vi "ParentModuleTemplate.vi"(11 "Module Config":T2={"Name"="Direct Drive Control System", "Parent Q"=refnum, "Is Child?"=FALSE, "Index"=0, "Dirs"={"Root"=path "", "Config"=path "C:/ATE/Config", "Logs"=path "C:/ATE/Logs", "Reports"=path "C:/ATE/Reports", "App Data"=path "C:/ProgramData/MAIN"}}) -> ()   [LabVIEW 2016]
uses:
  <vilib>/KATE/Queues/Queue Utils.lvlib
  <vilib>/KATE/Module/Module Utils.lvlib
  <vilib>/KATE/Module/Public/Action - Window Tasks.ctl
  <vilib>/KATE/Scheduler/Scheduler.lvlib
  <vilib>/KATE/Event Log/Event Log.lvlib
  <vilib>/KATE/Module/Public/Error Report.ctl
  <vilib>/KATE/Files/File Utils.lvlib
  <vilib>/Utility/miscctls.llb/LVRowAndColumnUnsignedTypeDef.ctl
  Controls & Typedefs/Log File Info.ctl
  Utils/Config/Save Control States/Save Control - Action.ctl
  <vilib>/KATE/Queues/Q.Element.ctl
  <vilib>/KATE/Module/Module Config.ctl
  <vilib>/KATE/Module/Public/SW Version Info.ctl
  <vilib>/KATE/Module/Module.Working Dirs.ctl
panel:
  in  "Main UI Tab":enum32{"Operate", "Maint"}(tab)
  in  "Main Ctrl Tab":enum32{"Page 1", "Page 2"}(tab)
  in  "Control1":bool
  in  "Test Name":string="TestX" caption="(Report name)"
  in  "Operator":string
  out "Rev":string="v0.0.1"
  out "Simulate Indication":string="Simulating Instruments"
  out "Error":bool
  out "Title":string="App Name"
  in  "Data Tab":T1(tab)
  in  "Setup Control1":bool
  in  "Log Interval(s)":dbl=1.0
  in  "Open Log Folder":bool
  out "Report File Name":string
  out "Data Log":string[][](table)
  in  "Equipment List":string[][](table)=[["Function Generator", "", "", "", ""], ["", "", "", "", ""], ["", "", "", "", ""], ["", "", "", "", ""], ["", "", "", "", ""]]
  in  "Reset":bool
  out "Status":string
  out "Test Ctrl Tab":enum32{"Idle", "Running", "Completed"}(tab)
  in  "Start":bool
  out "Status Duration(s)":dbl caption="Duration(s)" format="%.1f"
  out "Status Elapsed(s)":dbl caption="Elapsed(s)" format="%.1f"
  out "Test Running":bool
  out "Progress":dbl(slide) scale=0.0..1.0
  in  "Abort":bool
  in  "Test Reset":bool
  in  "Simulate En":bool
  in  "Exit":bool
  in  "Show Block Diagram":bool
  in  "Leave Maint":bool
  in  "Maint":bool
  in  "SW Rev":T4={"AppName"="App Name", "Company"="Company Name", "Version"="0.0.1", "Date"="xx/xx/xx"}
  # "Company Icon"
  # "Test Info"
  # "Put controls here that you want \nto be always visible"
  # "Put test setup controls here"
  # "This si a subpanel to a child VI that controls the instrument"
  # "Function Generator\nInternal Memory Status"
  # "<Update Version and save as default values>"
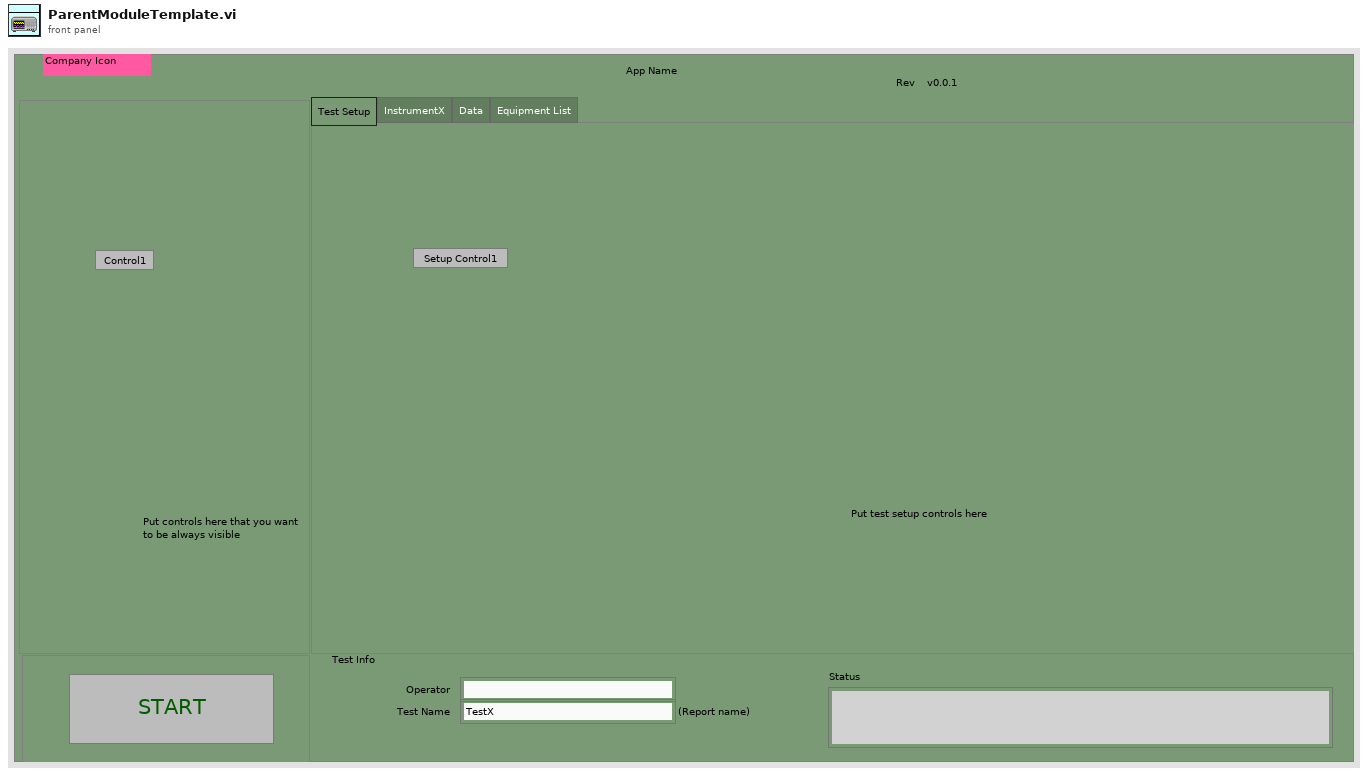
[diagram p1: front panel]
types:
  T1 = enum32{"Test Setup", "InstrumentX", "Data", "Equipment List"}
  T2 = typedef "KATE_Lib.lvlib/Module Utils.lvlib/Module Config.ctl" = cluster{"Name":string, "Parent Q":refnum<queue>, "Is Child?":bool, "Index":i32, "Dirs":T3}
  T3 = typedef "KATE_Lib.lvlib/Module Utils.lvlib/Module.Working Dirs.ctl" = cluster{"Root":path, "Config":path, "Logs":path, "Reports":path, "App Data":path}
  T4 = typedef "KATE_Lib.lvlib/Module Utils.lvlib/SW Version Info.ctl" = cluster{"AppName":string, "Company":string, "Version":string, "Date":string}
  T5 = typedef "KATE_Lib.lvlib/Module Utils.lvlib/Module Sys Info.ctl" = cluster{"Main Q":refnum<queue>, "Exe":bool, "SW Rev":T6, "Self Ref":refnum<vi>, "Main Tab":refnum<vi>, "Pane":refnum<vi>, "Stop":cluster{"Ref":refnum<event-registration>, "Event":refnum<user-event>}, "Cfg":T2, "Services":cluster{"Name":string, "vi ref":refnum<vi>}[]}
  T6 = typedef "KATE_Lib.lvlib/Module Utils.lvlib/Module.SW Version Info.ctl" = cluster{"AppName":string, "Company":string, "Version":string, "Date":string}
  T7 = typedef "KATE_Lib.lvlib/Module Utils.lvlib/Action - Window Tasks.ctl" = enum16{"Resize()", "Show Panel(Bool)", "Show Scroll Bars(Bool)", "Dock to SubPanel(SubPanel Ref)", "Undock from SubPanel()", "Return to SubPanel()", "Go To Maint Tab()", "Show Maint Tab(Bool)", "Open Block Diagram()"}
  T8 = cluster{"Test Start(s)":dbl, "StepStart(s)":dbl, "Running":bool}
  T9 = typedef "Save Control - Action.ctl" = enum16{"Read", "Save", "Add Single Ctrl", "Add Mult Ctrls", "Restore"}
  T10 = enum8{"Enabled", "Disabled", "Disabled and Grayed Out"}
  T11 = typedef "LVRowAndColumnUnsignedTypeDef.ctl" = cluster{"Row":u32, "Column":u32}
  T12 = typedef "Log File Info.ctl" = cluster{"Log Name":string, "Initialized":bool, "Cmt Flag":bool, "Open":bool, "FileRef":refnum<k34>}
  T13 = enum16{"open", "open or create", "create or replace", "create", "open (read-only)"}
  T14 = enum16{"Top Left", "Top Right", "Bottom Left", "Bottom Right"}
  T15 = cluster{"Test State":cluster{"Test Start(s)":dbl, "StepStart(s)":dbl, "Running":bool}, "Data Table":string[][], "Log":T12}
  T16 = typedef "KATE_Lib.lvlib/Module Utils.lvlib/Error Report.ctl" = cluster{"Cnt":i32, "Recent Error":errorcluster}
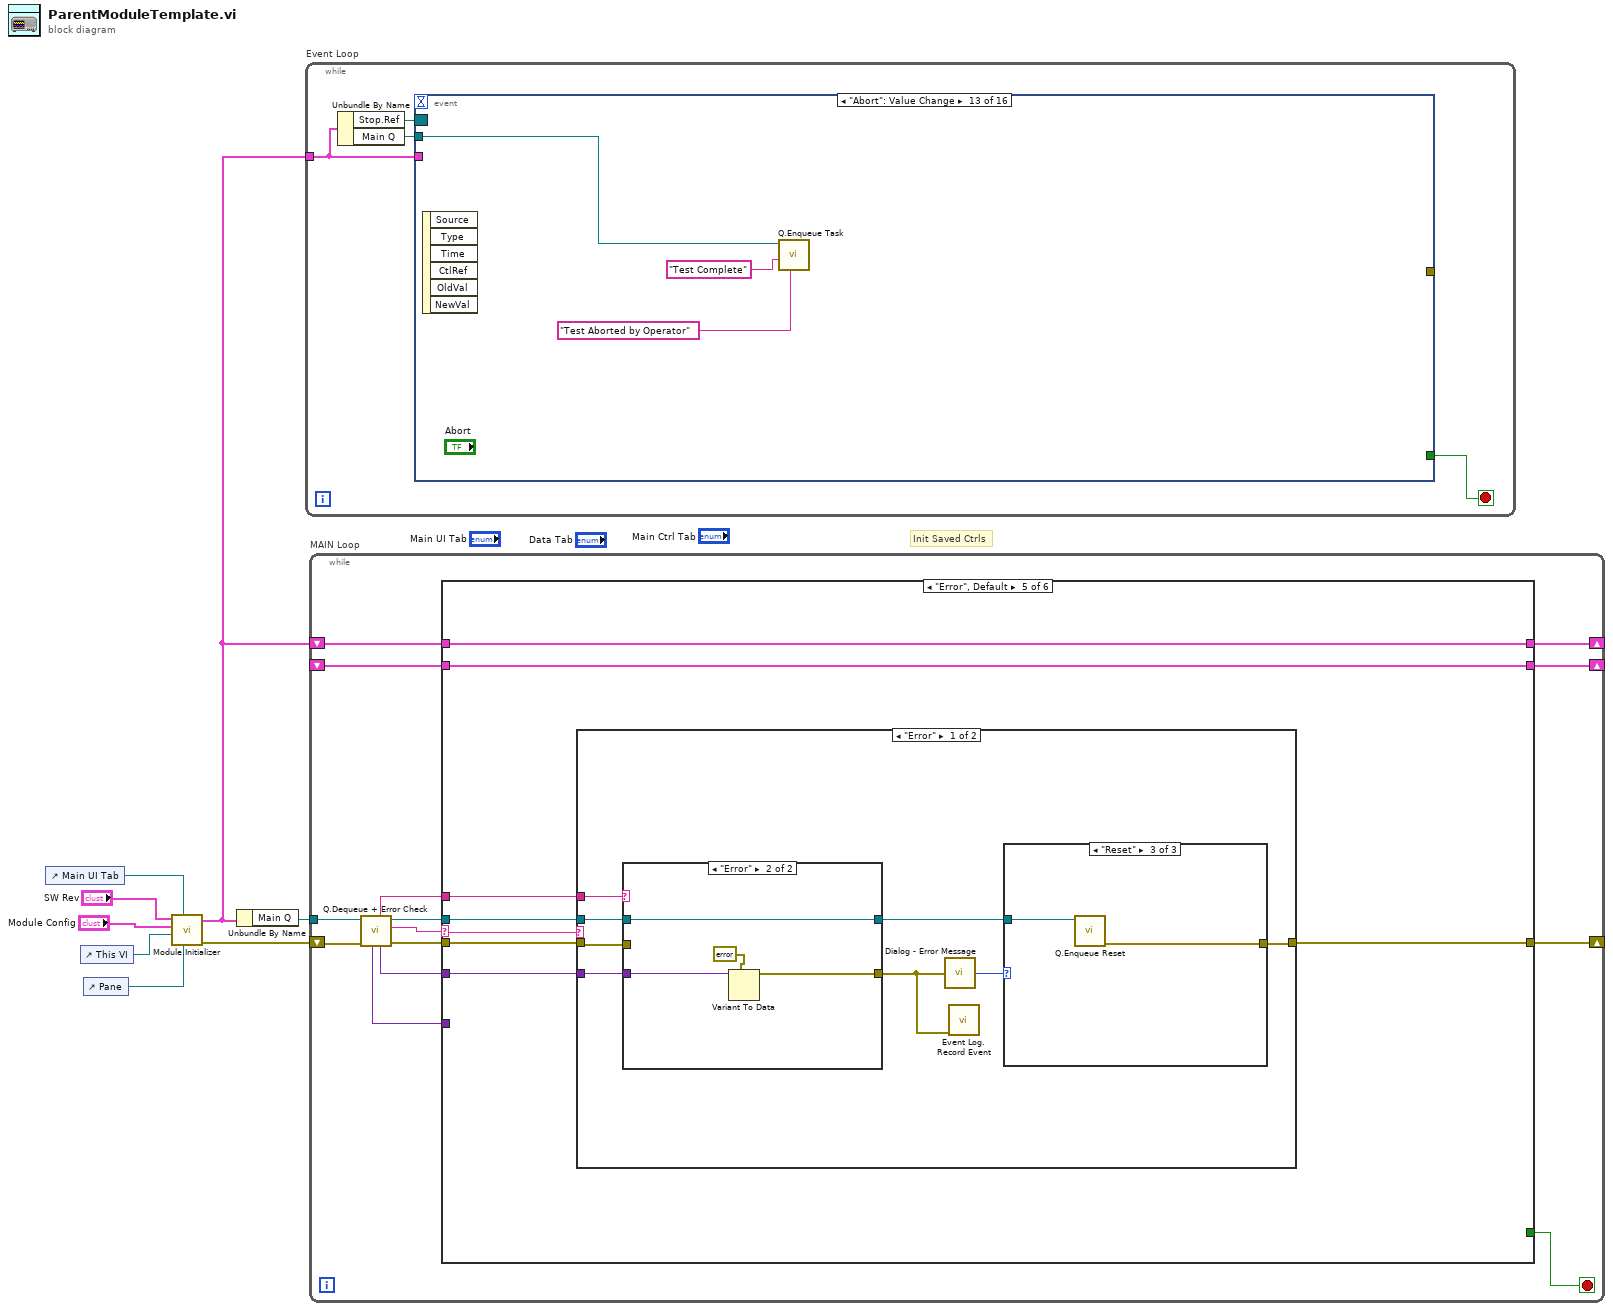
[diagram p0: block diagram]
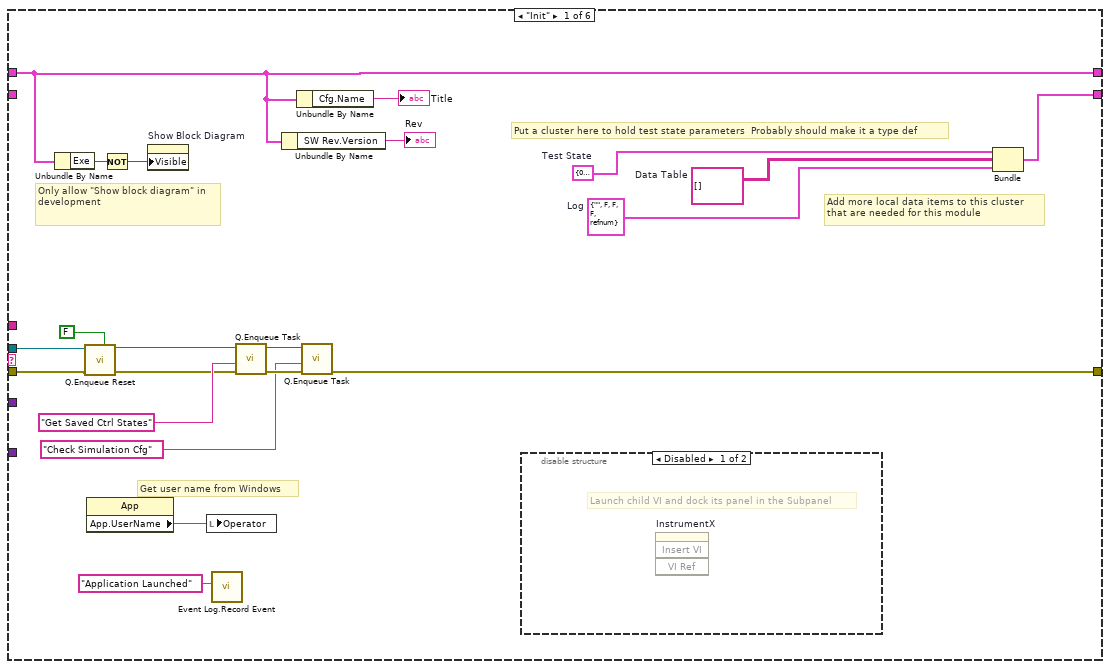
[diagram p2: hidden frame]
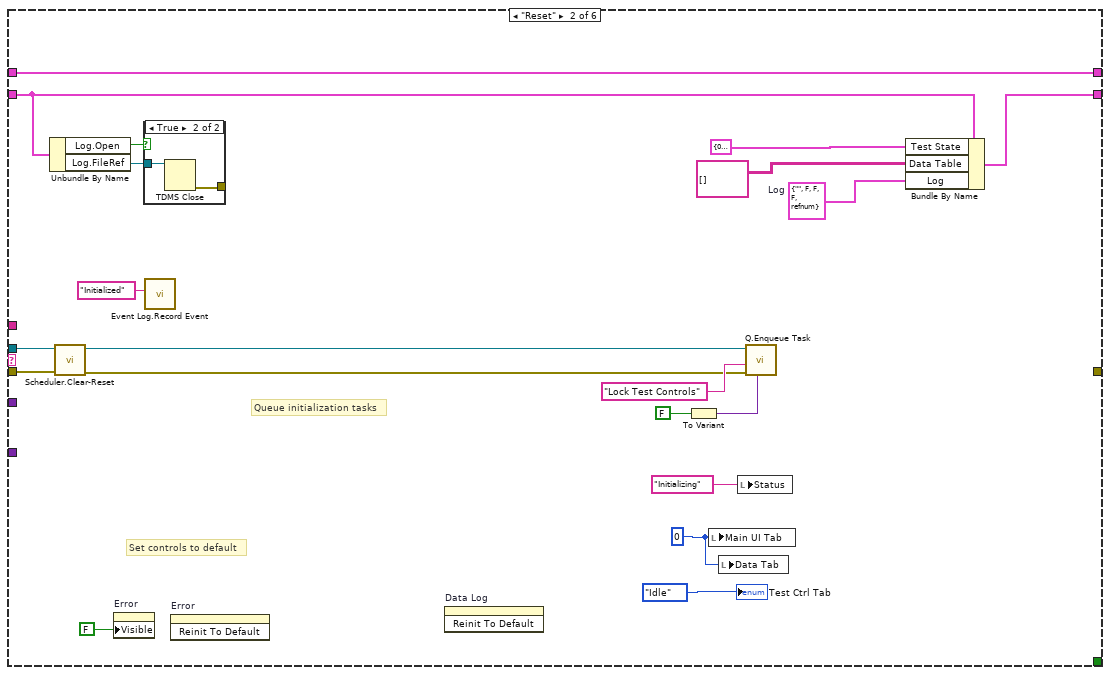
[diagram p4: hidden frame]
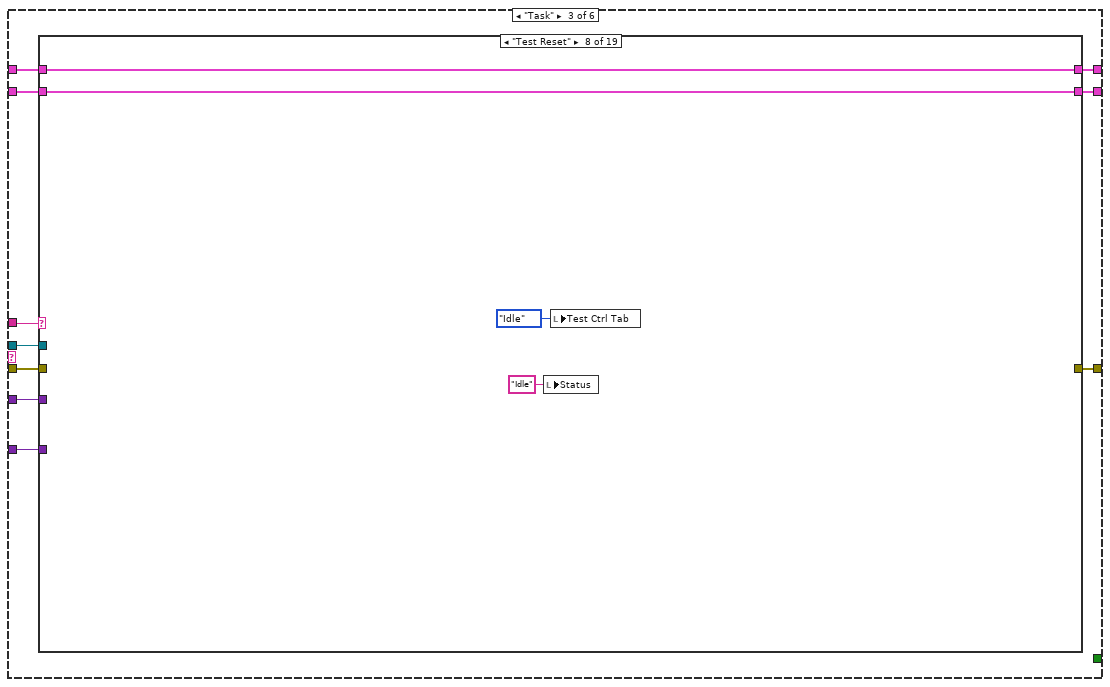
[diagram p6: hidden frame]
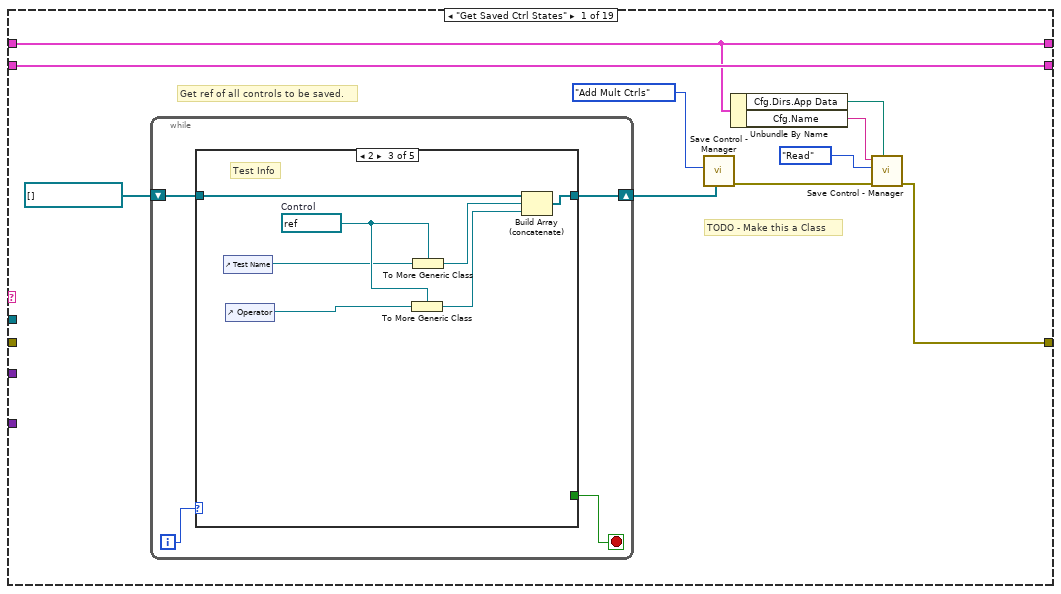
[diagram p7: hidden frame]
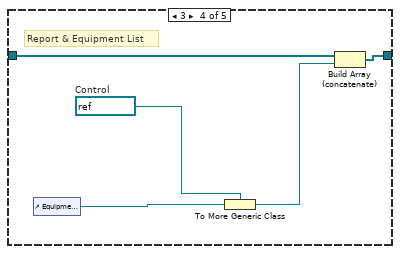
[diagram p10: hidden frame]
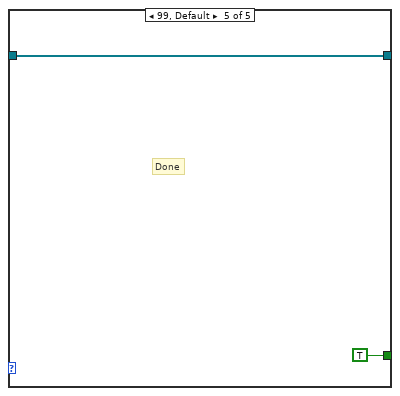
[diagram p11: hidden frame]
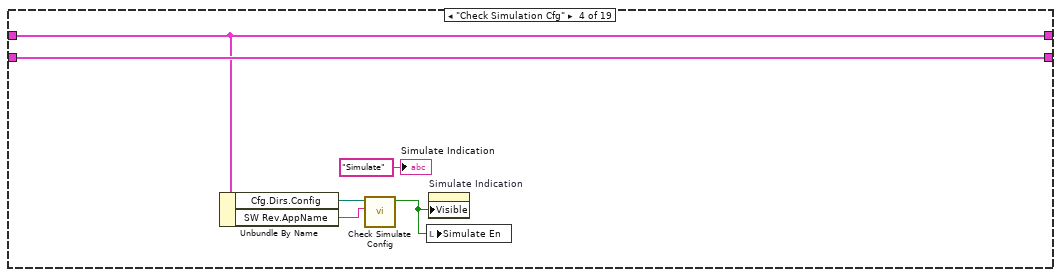
[diagram p14: hidden frame]
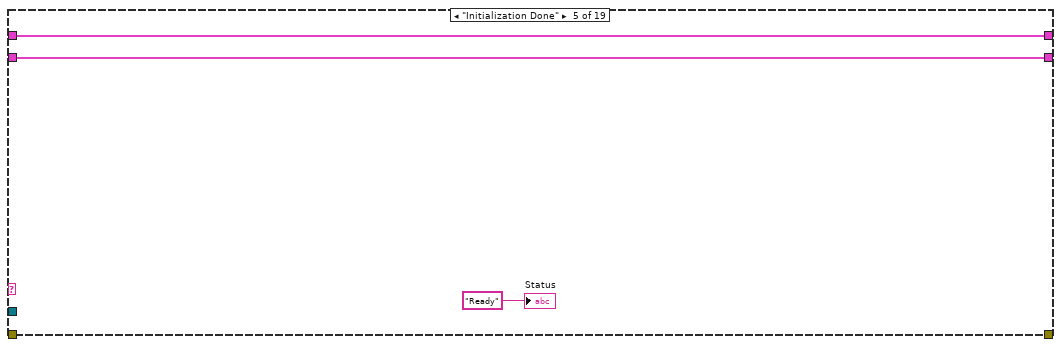
[diagram p15: hidden frame]
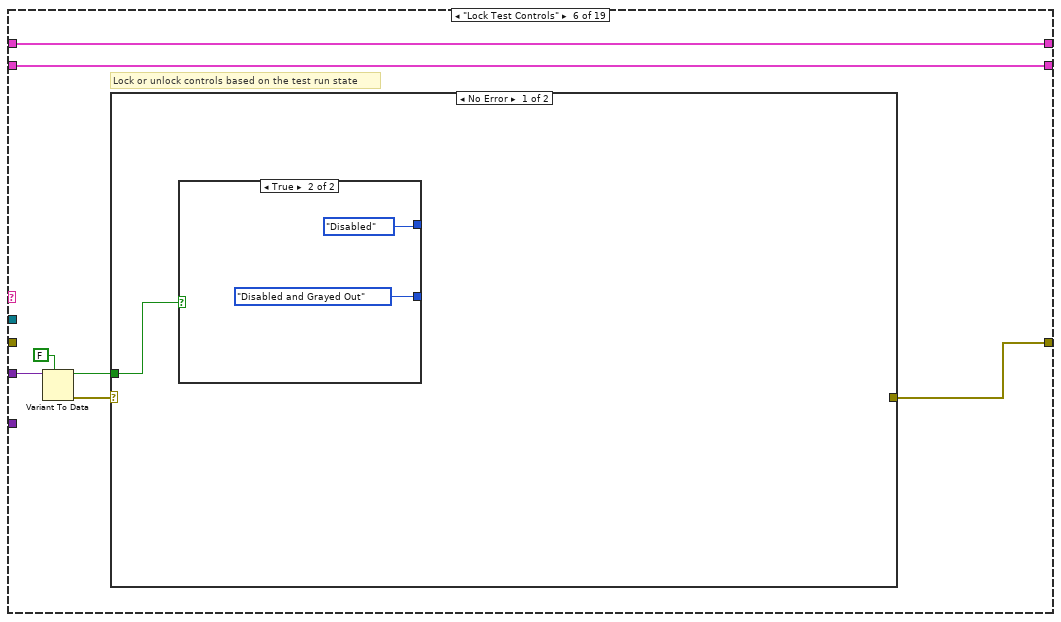
[diagram p16: hidden frame]
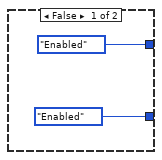
[diagram p17: hidden frame]
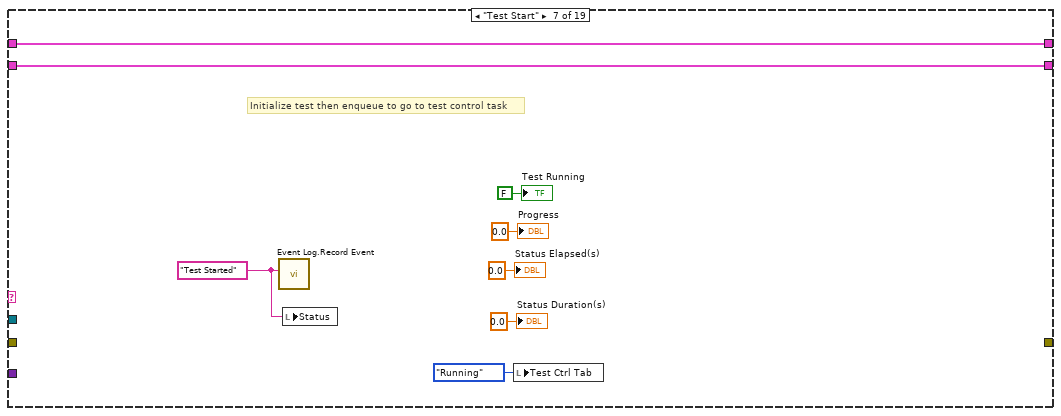
[diagram p19: hidden frame]
diagram:
  # "Init Saved Ctrls"
  n1 = control-ref of="Main UI Tab"() -> (w5:refnum<vi>)
  n2 = control-ref of="This VI"() -> (w4:refnum<vi>)
  n3 = control-ref of="Pane"() -> (w3:refnum<vi>)
  n4 = call <vilib>:"Module.Initializer.vi"("Pane"=w3, "Main Tab"=w5, "Self Ref"=w4, "Module Config"="Module Config", "SW Rev"="SW Rev") -> ("error out"=w8:errorcluster, "Sys"=w7:T5)  [unwired: 5 in]
  n5 = Unbundle By Name(w7) -> ("Main Q"=w6:refnum<queue>)
  n6 = while "Event Loop" {
    tunnel: w7 -> [w11]
    stop <- w12 stop-if-true
    n7 = Unbundle By Name(w11) -> ("Stop.Ref"=w10:refnum<event-registration>, "Main Q"=w9:refnum<queue>)
    n8 = event shown="[12] \"Abort\": Value Change" {
      selector: w10 -> [_ _ _ _ _ _ _ _ _ _ _ _ _ _ _ _]
      dyn-events: _ -> [_ _ _ _ _ _ _ _ _ _ _ _ _ _ _ _]
      timeout: _ -> [_ _ _ _ _ _ _ _ _ _ _ _ _ _ _ _]
      tunnel: [w16 TRUE _ _ _ _ _ w40 TRUE _ _ _ _ _ _ _] -> w12
      tunnel: w11 -> [w15 _ _ _ _ _ _ w38 _ w65 _ _ _ _ w81 _]
      tunnel: w9 -> [w18 w28 w30 w32 w34 w36 _ w39 _ _ w66 w71 w76 w78 _ w82]
      tunnel: [_ _ _ _ _ _ _ _ _ _ _ _ _ _ w79 _] -> _
      event Panel Close? {
        n9 = event-data() -> ()  [unwired: 1 in, 4 out]
        n10 = Unbundle By Name(w15) -> ("Exe"=w13:bool, "Cfg.Is Child?"=w14:bool)
        n11 = case shown="False" w14 {
          tunnel: w18 -> [w22 w25]
          tunnel: [w20 TRUE] -> w17
          tunnel: [TRUE FALSE] -> w16
          tunnel: [_ w23] -> _
          tunnel: w13 -> [w19 _]
          frame False {
            # "Parent - Exit"
            n12 = call <vilib>:"Q.Enqueue Exit.vi"("Q In"=w22) -> ()  [unwired: 9 in, 2 out]
            n13 = Not(x=w19) -> (.not. x?=w20:bool)
          }
          frame True {
            # "Child - Hide Panel"
            n14 = call <vilib>:"Q Window Task.vi"("Action"=Action_-_Window_Tasks."Return to SubPanel()", "Q In"=w25) -> ("error out"=w23:errorcluster)  [unwired: 8 in, 1 out]
          }
        }
        n15 = event-data("Discard?"=w17) -> ()  [unwired: 1 in, 1 out]
      }
      event "Exit": Value Change {
        n16 = event-data() -> ()  [unwired: 1 in, 6 out]
        n17 = call <vilib>:"Q.Enqueue Exit.vi"("Q In"=w28) -> ()  [unwired: 9 in, 2 out]
      }
      event "Reset": Value Change {
        n18 = event-data() -> ()  [unwired: 1 in, 6 out]
        n19 = call <vilib>:"Q.Enqueue Reset.vi"("Q In"=w30) -> ()  [unwired: 9 in, 2 out]
      }
      event Panel Resize {
        n20 = event-data() -> ()  [unwired: 1 in, 8 out]
        n21 = call <vilib>:"Q Window Task.vi"("Action"=Action_-_Window_Tasks."Resize()", "Q In"=w32) -> ()  [unwired: 8 in, 2 out]
      }
      event "Show Block Diagram": Value Change {
        n22 = event-data() -> ()  [unwired: 1 in, 6 out]
        n23 = call <vilib>:"Q Window Task.vi"("Action"=Action_-_Window_Tasks."Open Block Diagram()", "Q In"=w34) -> ()  [unwired: 8 in, 2 out]
      }
      event "Maint": Value Change {
        n24 = event-data() -> ()  [unwired: 1 in, 6 out]
        n25 = call <vilib>:"Q Window Task.vi"("Action"=Action_-_Window_Tasks."Go To Maint Tab()", "Q In"=w36) -> ()  [unwired: 8 in, 2 out]
      }
      event "Leave Maint": Value Change {
        n26 = event-data() -> ()  [unwired: 1 in, 6 out]
        n27 = local write "Main UI Tab"(0) -> ()
      }
      event Menu Selection (User) {
        n28 = event-data() -> ("ItemTag"=w41:string)  [unwired: 1 in, 6 out]
        n29 = case shown="Default" w41 {
          tunnel: [_ TRUE _ _ _ _ _] -> w40
          tunnel: w39 -> [_ w42 _ w45 _ _ _]
          tunnel: [_ _ w44 _ w46 _ w51] -> _
          tunnel: w38 -> [_ _ _ _ w47 w50 w60]
          frame Default {
          }
          frame "Exit" {
            n30 = call <vilib>:"Q.Enqueue Exit.vi"("Q In"=w42) -> ()  [unwired: 9 in, 2 out]
          }
          frame "Show Event Log" {
            n31 = call <vilib>:"Event Log.Show.vi"() -> ("error out"=w44:errorcluster)  [unwired: 11 in]
          }
          frame "Reset" {
            n32 = call <vilib>:"Q.Enqueue Reset.vi"("Q In"=w45) -> ()  [unwired: 9 in, 2 out]
          }
          frame "Open Log Folder" {
            n33 = Unbundle By Name(w47) -> ("Cfg.Dirs.Logs"=w48:path)
            n34 = call <vilib>:"File.Open File or Folder.vi"("Path"=w48) -> ("Error Out"=w46:errorcluster)  [unwired: 10 in]
          }
          frame "Help.About" {
            n35 = Unbundle By Name(w50) -> ("SW Rev"=w49:T6)
            n36 = call "Help.About.vi"("SW Version"=w49) -> ()  [unwired: 11 in]
          }
          frame "Help.User Manual" {
            n37 = Unbundle By Name(w60) -> ("SW Rev.AppName"=w59:string)
            n38 = call <vilib>:"Application Directory.vi"() -> ("Application Directory"=w55:path)
            n39 = Build Path(base path=w55, name or relative path="Documentation") -> (appended path=w54:path)
            n40 = Concatenate Strings("User Manual, ", w59, ".pdf") -> (w53:string)
            n41 = Build Path(base path=w54, name or relative path=w53) -> (appended path=w52:path)
            n42 = call <vilib>:"File.Open File or Folder.vi"("Path"=w52) -> ("Error Out"=w51:errorcluster)  [unwired: 10 in]
          }
        }
      }
      event User Event {
        n43 = event-data() -> ()  [unwired: 1 in, 5 out]
      }
      event "Simulate En": Value Change {
        n44 = event-data() -> ()  [unwired: 1 in, 6 out]
        n45 = Unbundle By Name(w65) -> ("Cfg.Dirs.Config"=w64:path, "SW Rev.AppName"=w63:string)
        n46 = call "Save Simulate Config.vi"("Simulate"="Simulate En", "App Name"=w63, "Config Folder"=w64) -> ()  [unwired: 8 in, 1 out]
        n47 = property on="Simulate Indication" class="Str"("Visible"="Simulate En") -> ()  [unwired: 2 in, 2 out]
      }
      event "Control1": Value Change {
        # "This code is a template for how to handle a control event.  \nEnque one or more tasks to handle the control change event"
        n48 = event-data() -> ()  [unwired: 1 in, 6 out]
        n49 = To Variant(anything="Control1") -> (Variant=w68:variant)
        n50 = call <vilib>:"Q.Enqueue Task.vi"("Data1"=w68, "Task Name"="Control1", "Q In"=w66) -> ()  [unwired: 7 in, 2 out]
      }
      event "Setup Control1": Value Change {
        # "This code is a template for how to handle a control event.  \nEnque one or more tasks to handle the control change event"
        n51 = event-data() -> ()  [unwired: 1 in, 6 out]
        n52 = To Variant(anything="Setup Control1") -> (Variant=w72:variant)
        n53 = call <vilib>:"Q.Enqueue Task.vi"("Data1"=w72, "Task Name"="Setup Control1", "Q In"=w71) -> ()  [unwired: 7 in, 2 out]
      }
      event "Abort": Value Change {
        n54 = event-data() -> ()  [unwired: 1 in, 6 out]
        n55 = call <vilib>:"Q.Enqueue Task.vi"("Data1"="Test Aborted by Operator" ("Message"), "Task Name"="Test Complete", "Q In"=w76) -> ()  [unwired: 7 in, 2 out]
      }
      event "Test Reset": Value Change {
        n56 = event-data() -> ()  [unwired: 1 in, 6 out]
        n57 = call <vilib>:"Q.Enqueue Task.vi"("Task Name"="Test Reset", "Q In"=w78) -> ()  [unwired: 8 in, 2 out]
      }
      event "Open Log Folder": Value Change {
        n58 = event-data() -> ()  [unwired: 1 in, 6 out]
        n59 = Unbundle By Name(w81) -> ("Cfg.Dirs.Reports"=w80:path)
        n60 = call <vilib>:"File.Open File or Folder.vi"("Path"=w80) -> ("Error Out"=w79:errorcluster)  [unwired: 10 in]
      }
      event "Start": Value Change {
        n61 = event-data() -> ()  [unwired: 1 in, 6 out]
        n62 = call <vilib>:"Q.Enqueue Task.vi"("Task Name"="Test Start", "Q In"=w82) -> ()  [unwired: 8 in, 2 out]
      }
    }
  }
  n63 = while "MAIN Loop" {
    shift-right: [w93] -> _
    shift-left: w8 -> [w91]
    shift-right: [w94] -> _
    shift-left: _ -> [w97]
    shift-right: [w95] -> _
    shift-left: w7 -> [w96]
    tunnel: w6 -> [w90]
    stop <- w84 stop-if-true
    n64 = call <vilib>:"Q.Dequeue + Error Check.vi"("Error In"=w91, "Q In"=w90) -> ("error out"=w92:errorcluster, "Cmd"=w89:string, "Q Out"=w88:refnum<queue>, "Data1"=w87:variant, "Sub"=w85:string, "Data2"=w86:variant)  [unwired: 4 in]
    n65 = case shown="\"Error\", Default" w89 {
      selector: w89 -> [_ _ _ _ w440 _]
      tunnel: w97 -> [_ w125 w149 w430 w442 w469]
      tunnel: w96 -> [w106 w131 w150 w431 w443 w471]
      tunnel: [w106 w131 w148 w429 w443 w471] -> w95
      tunnel: [w102 w133 w147 w428 w442 w469] -> w94
      tunnel: [w101 _ w141 w423 w441 w477] -> w93
      tunnel: w92 -> [w117 w137 w143 w424 w438 _]
      tunnel: w88 -> [w118 w138 w144 w425 w436 _]
      tunnel: w87 -> [_ _ w145 w426 w439 _]
      tunnel: w86 -> [_ _ w142 w422 _ _]
      tunnel: w85 -> [_ _ w146 w427 w437 _]
      tunnel: [_ _ _ _ _ TRUE] -> w84
      frame "Init" {
        w100 = T8 {"Test Start(s)"=0.0, "StepStart(s)"=0.0, "Running"=FALSE}  # Test State
        w108 = T12 {"Log Name"="", "Initialized"=FALSE, "Cmt Flag"=FALSE, "Open"=FALSE, "FileRef"=refnum}  # Log
        w112 = string[][] []  # Data Table
        # "Add more local data items to this cluster \nthat are needed for this module"
        # "Put a cluster here to hold test state parameters  Probably should make it a type def"
        # "Get user name from Windows"
        # "Only allow \"Show block diagram\" in development"
        n66 = Unbundle By Name(w106) -> ("Exe"=w115:bool)
        n67 = call <vilib>:"Q.Enqueue Reset.vi"("Top of Q(T)"=FALSE ("Flush Q"), "Error In"=w117, "Q In"=w118) -> ("error out"=w98:errorcluster, "Q Out"=w99:refnum<queue>)  [unwired: 7 in]
        n68 = property class="App"() -> ("App.UserName"=w109:string)  [unwired: 2 in, 2 out]
        n69 = Not(x=w115) -> (.not. x?=w114:bool)
        n70 = property on="Show Block Diagram" class="Bool"("Visible"=w114) -> ()  [unwired: 2 in, 2 out]
        n71 = local write "Operator"(w109) -> ()
        n72 = call <vilib>:"Event Log.Record Event.vi"("Message"="Application Launched") -> ()  [unwired: 10 in, 1 out]
        n73 = call <vilib>:"Q.Enqueue Task.vi"("Error In"=w98, "Task Name"="Get Saved Ctrl States", "Q In"=w99) -> ("error out"=w104:errorcluster, "Q Out"=w105:refnum<queue>)  [unwired: 7 in]
        n74 = Unbundle By Name(w106) -> ("SW Rev.Version"=→"Rev":string)
        n75 = Unbundle By Name(w106) -> ("Cfg.Name"=→"Title":string)
        n76 = call <vilib>:"Q.Enqueue Task.vi"("Error In"=w104, "Task Name"="Check Simulation Cfg", "Q In"=w105) -> ("error out"=w101:errorcluster)  [unwired: 7 in, 1 out]
        n77 = disable-structure shown="Disabled" {
          frame Disabled {
            # "Launch child VI and dock its panel in the Subpanel"
            n78 = invoke on="InstrumentX" class="SubPnl" method="Insert VI"() -> ()  [unwired: 4 in, 4 out]
          }
          frame Enabled {
          }
        }
        n79 = Bundle("Test State"=w100, "Data Table"=w112, "Log"=w108) -> (w102:T15)  [unwired: 1 in]
      }
      frame "Reset" {
        w126 = T12 {"Log Name"="", "Initialized"=FALSE, "Cmt Flag"=FALSE, "Open"=FALSE, "FileRef"=refnum}  # Log
        w134 = 0
        # "Set controls to default"
        # "Queue initialization tasks"
        n80 = Unbundle By Name(w125) -> ("Log.Open"=w123:bool, "Log.FileRef"=w124:refnum<k34>)
        n81 = call <vilib>:"Scheduler.Clear-Reset.vi"("error in"=w137, "Q In"=w138) -> ("error out"=w120:errorcluster, "Q Out"=w119:refnum<queue>)  [unwired: 8 in]
        n82 = property on="Error" class="Bool (strict)"("Visible"=FALSE) -> ()  [unwired: 2 in, 2 out]
        n83 = case shown="True" w123 {
          tunnel: w124 -> [_ w140]
          tunnel: [_ w139] -> _
          frame False {
          }
          frame True {
            n84 = TDMS Close(11:w140) -> (0:w139:errorcluster)  [unwired: 1 in, 1 out]
          }
        }
        n85 = call <vilib>:"Event Log.Record Event.vi"("Message"="Initialized") -> ()  [unwired: 10 in, 1 out]
        n86 = invoke on="Error" class="Bool (strict)" method="Reinit To Default"() -> ()  [unwired: 3 in, 3 out]
        n87 = invoke on="Data Log" class="Tbl (strict)" method="Reinit To Default"() -> ()  [unwired: 3 in, 3 out]
        n88 = To Variant(anything=FALSE) -> (Variant=w129:variant)
        n89 = local write "Main UI Tab"(w134) -> ()
        n90 = local write "Data Tab"(w134) -> ()
        n91 = local write "Status"("Initializing" ("Status")) -> ()
        n92 = call <vilib>:"Q.Enqueue Task.vi"("Data1"=w129, "Error In"=w120, "Task Name"="Lock Test Controls", "Q In"=w119) -> ()  [unwired: 6 in, 2 out]
        n93 = Bundle By Name(cluster=w125, "Test State"=T8 {"Test Start(s)"=0.0, "StepStart(s)"=0.0, "Running"=FALSE}, "Data Table"=string[][] [], "Log"=w126) -> (w133:T15)
        "Test Ctrl Tab" <- enum32{"Idle", "Running", "Completed"}."Idle" ("Test Ctrl Tab")
      }
      frame "Task" {
        n94 = case shown="\"Test Reset\"" w146 {
          selector: w146 -> [_ _ _ _ _ _ _ _ _ _ _ _ _ _ _ _ _ _ w417]
          tunnel: w150 -> [w153 w182 w184 w185 w193 w200 w214 w218 w220 w228 w244 w256 w301 w334 w371 w381 w388 w391 w418]
          tunnel: w149 -> [w160 w181 w183 w190 w192 w199 w213 w217 w219 w227 w233 w258 w299 w331 w366 w380 w387 w392 w419]
          tunnel: [w153 w182 w184 w185 w193 w200 w214 w218 w220 w228 w244 w256 w301 w334 w371 w381 w388 w391 w418] -> w148
          tunnel: [w160 w181 w183 w190 w192 w199 w213 w217 w219 w227 w238 w257 w298 w331 w366 w379 w387 w392 w419] -> w147
          tunnel: w145 -> [_ _ _ _ _ w198 _ _ _ w225 _ _ _ _ w370 _ w386 _ w416]
          tunnel: w144 -> [_ _ _ _ _ _ _ _ _ _ w232 w262 _ w332 _ _ _ _ _]
          tunnel: w143 -> [_ _ _ _ _ _ _ _ _ _ _ _ _ _ _ _ _ _ w414]
          tunnel: w142 -> [_ _ _ _ _ _ _ _ _ _ _ _ _ _ _ _ _ _ w415]
          tunnel: [w151 _ _ _ _ w194 _ _ _ _ _ w249 w293 _ w361 _ _ _ w413] -> w141
          frame "Get Saved Ctrl States" {
            # "TODO - Make this a Class"
            # "Get ref of all controls to be saved."
            n95 = while {
              shift-right: [w162] -> w157
              shift-left: refnum<vi>[] [] -> [w163]
              i -> [w164]
              stop <- w161 stop-if-true
              n96 = case shown="2" w164 {
                tunnel: w163 -> [w165 w166 w172 w177 w180]
                tunnel: [w165 w166 w173 w178 w180] -> w162
                tunnel: [_ _ _ _ TRUE] -> w161
                frame 0 {
                  # "Setup Controls"
                }
                frame 1 {
                  # "Main Controls"
                }
                frame 2 {
                  w171 = refnum<vi> refnum  # Control
                  # "Test Info"
                  n97 = control-ref of="Test Name"() -> (w168:refnum<vi>)
                  n98 = control-ref of="Operator"() -> (w167:refnum<vi>)
                  n99 = To More Generic Class(target class=w171, reference=w167) -> (generic class reference=w169:refnum<vi>)
                  n100 = To More Generic Class(target class=w171, reference=w168) -> (generic class reference=w170:refnum<vi>)
                  n101 = Build Array (concatenate)(w172, w170, w169) -> (w173:refnum<vi>[])
                }
                frame 3 {
                  w175 = refnum<vi> refnum  # Control
                  # "Report & Equipment List"
                  n102 = control-ref of="Equipment List"() -> (w174:refnum<vi>)
                  n103 = To More Generic Class(target class=w175, reference=w174) -> (generic class reference=w176:refnum<vi>)
                  n104 = Build Array (concatenate)(w177, w176) -> (w178:refnum<vi>[])
                }
                frame 99, Default {
                  # "Done"
                }
              }
            }
            n105 = call "Save Control - Manager.vi"("Ctrl Array"=w157, "Action"=Save_Control_-_Action."Add Mult Ctrls") -> ("error out"=w152:errorcluster)  [unwired: 9 in]
            n106 = Unbundle By Name(w153) -> ("Cfg.Dirs.App Data"=w154:path, "Cfg.Name"=w155:string)
            n107 = call "Save Control - Manager.vi"("App Data Dir"=w154, "error in"=w152, "Action"=Save_Control_-_Action."Read", "App Name"=w155) -> ("error out"=w151:errorcluster)  [unwired: 7 in]
          }
          frame "Setup Control1" {
            # "Handle Setup Control state change"
          }
          frame "Control1" {
            # "Handle Control state change"
          }
          frame "Check Simulation Cfg" {
            n108 = Unbundle By Name(w185) -> ("Cfg.Dirs.Config"=w189:path, "SW Rev.AppName"=w188:string)
            n109 = call "Check Simulate Config.vi"("App Name"=w188, "Config Folder"=w189) -> ("Simulate"=w186:bool)  [unwired: 9 in]
            n110 = local write "Simulate En"(w186) -> ()
            n111 = property on="Simulate Indication" class="Str"("Visible"=w186) -> ()  [unwired: 2 in, 2 out]
            "Simulate Indication" <- "Simulate" ("Simulate Indication")
          }
          frame "Initialization Done" {
            "Status" <- "Ready" ("Status")
          }
          frame "Lock Test Controls" {
            # "Lock or unlock controls based on the test run state"
            n112 = Variant To Data(type=FALSE, Variant=w198) -> (data=w195:bool, error out=w196:errorcluster)  [unwired: 1 in]
            n113 = case shown="No Error" w196 {
              selector: w196 -> [_ w206]
              tunnel: w195 -> [w201 _]
              tunnel: [_ w206] -> w194
              frame No Error {
                n114 = case shown="True" w201 {
                  tunnel: [T10."Enabled" ("Disabled") T10."Disabled and Grayed Out" ("Disabled")] -> _
                  tunnel: [T10."Enabled" ("Disabled") T10."Disabled" ("Disabled")] -> _
                  frame False {
                  }
                  frame True {
                  }
                }
              }
              frame Error {
              }
            }
          }
          frame "Test Start" {
            w207 = "Test Started" ("Message")
            # "Initialize test then enqueue to go to test control task"
            n115 = call <vilib>:"Event Log.Record Event.vi"("Message"=w207) -> ()  [unwired: 10 in, 1 out]
            n116 = local write "Status"(w207) -> ()
            n117 = local write "Test Ctrl Tab"(enum32{"Idle", "Running", "Completed"}."Running" ("Test Ctrl Tab")) -> ()
            "Progress" <- 0.0 ("Progress")
            "Status Elapsed(s)" <- 0.0 ("Status Elapsed(s)")
            "Status Duration(s)" <- 0.0 ("Status Duration(s)")
            "Test Running" <- FALSE ("Test Running")
          }
          frame "Test Reset" {
            n118 = local write "Status"("Idle" ("Status")) -> ()
            n119 = local write "Test Ctrl Tab"(enum32{"Idle", "Running", "Completed"}."Idle" ("Test Ctrl Tab")) -> ()
          }
          frame "Test Abort" {
          }
          frame "Test Complete" {
            n120 = Variant To Data(type="", Variant=w225) -> (data=w222:string)  [unwired: 1 in, 1 out]
            n121 = Concatenate Strings("Test Completed: " ("Message"), w222) -> (w221:string)
            n122 = local write "Test Ctrl Tab"(enum32{"Idle", "Running", "Completed"}."Completed" ("Test Ctrl Tab")) -> ()
            n123 = call <vilib>:"Event Log.Record Event.vi"("Message"=w221) -> ()  [unwired: 10 in, 1 out]
            n124 = local write "Status"(w221) -> ()
          }
          frame "Init Logging" {
            n125 = Unbundle By Name(w233) -> ("Log.Open"=w230:bool, "Log.FileRef"=w234:refnum<k34>)
            n126 = case shown="True" w230 {
              tunnel: w234 -> [_ w246]
              tunnel: [_ w245] -> _
              frame False {
              }
              frame True {
                n127 = TDMS Close(11:w246) -> (0:w245:errorcluster)  [unwired: 1 in, 1 out]
              }
            }
            n128 = call <vilib>:"Q.Enqueue Task.vi"("Task Name"="Init Log File", "Q In"=w232) -> ()  [unwired: 8 in, 2 out]
            n129 = Format Date/Time String(time format string (%c)="%Y-%m-%d_%H-%M-%S") -> (date/time string=w240:string)  [unwired: 2 in]
            n130 = property on="Data Log" class="Tbl (strict)"("Index Values"=T11 {"Row"=0, "Column"=0}) -> ()  [unwired: 2 in, 2 out]
            n131 = Concatenate Strings("Test Name", ", ", w240, ".tdms") -> (w235:string)
            "Report File Name" <- w235
            n132 = Bundle By Name(cluster=T12 {"Log Name"="", "Initialized"=FALSE, "Cmt Flag"=FALSE, "Open"=FALSE, "FileRef"=refnum} ("Log"), "Log Name"=w235) -> (w236:T12)
            n133 = Bundle By Name(cluster=w233, "Log"=w236) -> (w238:T15)
          }
          frame "Init Log File" {
            n134 = Unbundle By Name(w258) -> ("Log"=w260:T12, "Test State.Running"=w247:bool)
            n135 = case shown="False" w247 {
              tunnel: w262 -> [w269 w288]
              tunnel: "Log Data" ("Sched Name") -> [w268 w287]
              tunnel: w260 -> [w267 w285]
              tunnel: [w263 w286] -> w259
              tunnel: w256 -> [_ w284]
              tunnel: [_ w275] -> w250
              tunnel: [_ w273] -> w255
              frame False {
                n136 = Unbundle By Name(w267) -> ("Open"=w265:bool, "FileRef"=w266:refnum<k34>)
                n137 = case shown="True" w265 {
                  tunnel: w266 -> [_ w271]
                  tunnel: [_ w270] -> _
                  frame False {
                  }
                  frame True {
                    n138 = TDMS Close(11:w271) -> (0:w270:errorcluster)  [unwired: 1 in, 1 out]
                  }
                }
                n139 = call <vilib>:"Scheduler.Delete Task.vi"("Sched Name"=w268, "Q In"=w269) -> ()  [unwired: 8 in, 2 out]
                n140 = Bundle By Name(cluster=w267, "Open"=FALSE) -> (w263:T12)
              }
              frame True {
                n141 = Unbundle By Name(w284) -> ("Cfg.Dirs.Reports"=w283:path)
                n142 = Unbundle By Name(w285) -> ("Log Name"=w282:string, "Initialized"=w277:bool)
                n143 = call <vilib>:"Scheduler.AddTask.vi"("Recurring"=TRUE, "Interval(s)"="Log Interval(s)", "Task Name"=w287, "Sched Name"=w287, "Q In"=w288) -> ("Q Out"=w279:refnum<queue>)  [unwired: 5 in, 1 out]
                n144 = Build Path(base path=w283, name or relative path=w282) -> (appended path=w273:path)
                n145 = TDMS Open(5:FALSE ("create index file? (T)"), 10:T13."open or create" ("operation (0:open)"), 11:w273) -> (0:w275:errorcluster, 3:w281:refnum<k34>)  [unwired: 4 in]
                n146 = case shown="False" w277 {
                  tunnel: w279 -> [w291 _]
                  tunnel: "Write Setup Info to Log File" ("Sched Name") -> [w290 _]
                  frame False {
                    n147 = call <vilib>:"Q.Enqueue Task.vi"("Task Name"=w290, "Q In"=w291) -> ()  [unwired: 8 in, 2 out]
                  }
                  frame True {
                  }
                }
                n148 = Bundle By Name(cluster=w285, "FileRef"=w281, "Open"=TRUE) -> (w286:T12)
              }
            }
            n149 = Path To String(path=w255) -> (string=w248:string)
            n150 = Bundle By Name(cluster=w258, "Log"=w259) -> (w257:T15)
            n151 = Concatenate Strings("Error opening log file \"" ("Error Desc"), w248, "\".  Verify:\n1. The file is not opened in another applicaiton (like Excel) where it is locked and cannot be opened by this application." ("Error Desc")) -> (w254:string)
            n152 = call "Error - Add Local Description.vi"("error in"=w250, "Error Code"=-5004, "Error Desc"=w254) -> ("error out"=w249:errorcluster)  [unwired: 8 in]
          }
          frame "Write Setup Info to Log File" {
            n153 = Unbundle By Name(w299) -> ("Log.FileRef"=w300:refnum<k34>)
            n154 = while {
              tunnel: [w306] -> w292
              shift-right: [w303] -> w296
              shift-left: w300 -> [w304]
              i -> [w305]
              stop <- w307 stop-if-true
              n155 = case shown="0" w305 {
                tunnel: [_ w323 w330] -> w306
                tunnel: w304 -> [w309 w314 w328]
                tunnel: [w309 w313 w327] -> w303
                tunnel: [TRUE _ _] -> w302
                frame 99, Default {
                }
                frame 0 {
                  # "Other Setup Info??"
                  n156 = local read "Test Name"() -> (w320:string)
                  n157 = Build Array(w320, "Operator") -> (w317:string[])
                  n158 = Build Array(string[] ["Test Name", "Operator", "Catheter SN", "Catheter SN", "Protocol Name"], w317) -> (w316:string[][])
                  n159 = Transpose 2D Array(2D array=w316) -> (transposed array=w315:string[][])
                  n160 = Build Array (concatenate)(w315, string[][] [] ("array")) -> (w312:string[][])
                  n161 = Transpose 2D Array(2D array=w312) -> (transposed array=w311:string[][])
                  n162 = TDMS Write(0:w314, 5:"Setup", 7:string[] ["Value", "Parameter"], 9:w311) -> (4:w313:refnum<k34>, 15:w323:errorcluster)  [unwired: 2 in, 2 out]
                }
                frame 1 {
                  n163 = property on="Equipment List" class="Tbl (strict)"() -> ("Column Headers[]"=w326:string[])  [unwired: 2 in, 2 out]
                  n164 = Transpose 2D Array(2D array="Equipment List") -> (transposed array=w324:string[][])
                  n165 = TDMS Write(0:w328, 5:"Equipment", 7:w326, 9:w324) -> (4:w327:refnum<k34>, 15:w330:errorcluster)  [unwired: 2 in, 2 out]
                }
              }
              n166 = Or(x=w306, y=w302) -> (x .or. y?=w307:bool)
            }
            n167 = Bundle By Name(cluster=w299, "Log.Initialized"=TRUE, "Log.FileRef"=w296) -> (w298:T15)
            n168 = call "Error - Add Local Description.vi"("error in"=w292, "Error Code"=-5004, "Error Desc"="Error writing to log file.  Verify:\n1. The file is not opened in another applicaiton (like Excel) where it is locked and cannot be opened by this application.") -> ("error out"=w293:errorcluster)  [unwired: 8 in]
          }
          frame "Log Data" {
            n169 = Unbundle By Name(w331) -> ("Test State.Running"=w333:bool)
            n170 = case shown="True" w333 {
              tunnel: w331 -> [_ w336]
              tunnel: w332 -> [_ w335]
              frame False {
              }
              frame True {
                n171 = stacked-sequence {
                  seq-local: [w337 _ _] -> [_ _ w356]
                  tunnel: w336 -> [w338 _ _]
                  tunnel: w335 -> [_ _ w357]
                  frame #0 {
                    w339 = "0"
                    # "Append Data to Table"
                    # "Put Data Here"
                    n172 = Unbundle By Name(w338) -> ("Test State.Test Start(s)"=w345:dbl)
                    n173 = call <vilib>:"High Resolution Relative Seconds.vi"() -> ("relative seconds"=w344:dbl)
                    n174 = Subtract(x=w344, y=w345) -> (x-y=w343:dbl)
                    n175 = Number To Fractional String(number=w343, precision (6)=i16 3) -> (F-format string=w341:string)  [unwired: 2 in]
                    n176 = Build Array(w341, w339, w339, w339, w339, w339, w339, w339, w339) -> (w337:string[])
                    n177 = local read "Data Log"() -> (w346:string[][])
                    n178 = Build Array (concatenate)(w346, w337) -> (→"Data Log":string[][])
                  }
                  frame #1 {
                    w351 = 22  # Rows displayed
                    # "Auto Scroll Table Row position"
                    n179 = local read "Data Log"() -> (w348:string[][])
                    n180 = Array Size(array=w348) -> (size(s)=w347:i32[])
                    n181 = Index Array(array=w347) -> (element=w352:i32)  [unwired: 1 in]
                    n182 = Subtract(x=w352, y=w351) -> (x-y=w350:i32)
                    n183 = Greater Than 0?(x=w350) -> (x > 0?=w349:bool)
                    n184 = case shown="True" w349 {
                      tunnel: w350 -> [_ w353]
                      frame False {
                      }
                      frame True {
                        n185 = Bundle By Name(cluster=T11 {"Row"=0, "Column"=0} ("Index Values"), "Row"=w353) -> (w355:T11)
                        n186 = property on="Data Log" class="Tbl (strict)"("Index Values"=w355) -> ()  [unwired: 2 in, 2 out]
                      }
                    }
                  }
                  frame #2 {
                    # "Append Data to file"
                    n187 = To Variant(anything=w356) -> (Variant=w358:variant)
                    n188 = call <vilib>:"Q.Enqueue Task.vi"("Data1"=w358, "Task Name"="Write to Log File", "Q In"=w357) -> ()  [unwired: 7 in, 2 out]
                  }
                }
              }
            }
          }
          frame "Write to Log File" {
            n189 = Variant To Data(type=string[] [], Variant=w370) -> (data=w368:string[])  [unwired: 1 in, 1 out]
            n190 = Build Array(w368) -> (w367:string[][])
            n191 = Unbundle By Name(w366) -> ("Log.Open"=w364:bool, "Log.FileRef"=w365:refnum<k34>)
            n192 = case shown="True" w364 {
              tunnel: w367 -> [_ w373]
              tunnel: w365 -> [_ w375]
              tunnel: [_ w374] -> w360
              frame False {
              }
              frame True {
                n193 = property on="Data Log" class="Tbl (strict)"() -> ("Column Headers[]"=w376:string[])  [unwired: 2 in, 2 out]
                n194 = Transpose 2D Array(2D array=w373) -> (transposed array=w372:string[][])
                n195 = TDMS Write(0:w375, 5:"Data", 7:w376, 9:w372) -> (15:w374:errorcluster)  [unwired: 2 in, 3 out]
              }
            }
            n196 = call "Error - Add Local Description.vi"("error in"=w360, "Error Code"=-5004, "Error Desc"="Error writing to log file.  Verify:\n1. The file is not opened in another applicaiton (like Excel) where it is locked and cannot be opened by this application.") -> ("error out"=w361:errorcluster)  [unwired: 8 in]
          }
          frame "Set Comment Flag" {
            n197 = Bundle By Name(cluster=w380, "Log.Cmt Flag"=TRUE) -> (w379:T15)
          }
          frame "Error Update" {
            w385 = T16 {"Cnt"=0, "Recent Error"={"status"=FALSE, "code"=0, "source"=""}}  # Error Report
            n198 = Variant To Data(type=w385, Variant=w386) -> (data=w384:T16)  [unwired: 1 in, 1 out]
            n199 = Unbundle By Name(w384) -> ("Cnt"=w383:i32)  [unwired: 1 out]
            n200 = Greater Than 0?(x=w383) -> (x > 0?=→"Error":bool)
          }
          frame "Resize" {
            n201 = Unbundle By Name(w391) -> ("Main Tab"=w390:refnum<vi>)
            n202 = control-ref of="Title"() -> (w389:refnum<vi>)
            n203 = while {
              tunnel: w390 -> [w394]
              tunnel: w389 -> [w393]
              i -> [w396]
              stop <- w395 stop-if-true
              n204 = case shown="0" w396 {
                tunnel: [_ TRUE] -> w395
                tunnel: w394 -> [w405 w411]
                tunnel: w393 -> [w397 w410]
                tunnel: [_ w408] -> _
                frame 0 {
                  n205 = property class="TabCtl"(reference=w405) -> ("Width"=w402:u32)  [unwired: 1 in, 2 out]
                  n206 = property class="Str"(reference=w397) -> ("Width"=w401:u32)  [unwired: 1 in, 2 out]
                  n207 = Subtract(x=w402, y=w401) -> (x-y=w400:u32)
                  n208 = Divide(x=w400, y=2) -> (x/y=w399:dbl)
                  n209 = To Long Integer(number=w399) -> (32bit integer=w398:i32)
                  n210 = call <vilib>:"Resize Util - Align Ctrl within Tab Ctrl.vi"("Child Ref Pos"=T14."Top Left", "dY"=10 ("dX"), "Parent Ref Pos"=T14."Top Left", "dX"=w398, "Child Ctrl"=w397, "Parent Tab Ctrl"=w405) -> ()  [unwired: 3 in, 3 out]
                }
                frame Default {
                  # "Done"
                  n211 = Build Array(w411, w410) -> (w409:refnum<vi>[])
                  n212 = Close Reference(reference=w409) -> (error out=w408:errorcluster)  [unwired: 1 in]
                }
              }
            }
          }
          frame Default {
            n213 = call <vilib>:"Module.Default Tasks.vi"("Sys"=w418, "error in"=w414, "Data2"=w415, "Data1"=w416, "Sub"=w417) -> ("error out"=w413:errorcluster)  [unwired: 6 in]
          }
        }
      }
      frame "Function" {
        n214 = case shown="Default" w427 {
          tunnel: w431 -> [w434]
          tunnel: w430 -> [w435]
          tunnel: [w434] -> w429
          tunnel: [w435] -> w428
          tunnel: w426 -> [_]
          tunnel: w425 -> [_]
          tunnel: w424 -> [w432]
          tunnel: w422 -> [_]
          tunnel: [w432] -> w421
          tunnel: [variant] -> w420
          frame Default {
            # "Do nothing.  The sender of the command will report an error (timeout or incorrect data)."
          }
        }
        n215 = call <vilib>:"Q.Return Function Data.vi"("error in"=w421, "Data2"=w422, "Ret Data"=w420) -> ("error out"=w423:errorcluster)  [unwired: 8 in]
      }
      frame "Error", Default {
        n216 = case shown="\"Error\"" w440 {
          selector: w440 -> [_ w462]
          tunnel: [w445 w463] -> w441
          tunnel: w439 -> [w451 _]
          tunnel: w438 -> [w449 _]
          tunnel: w437 -> [w450 _]
          tunnel: w436 -> [w447 _]
          frame "Error" {
            n217 = case shown="\"Error\"" w450 {
              tunnel: w451 -> [_ w461]
              tunnel: w449 -> [w457 _]
              tunnel: [w457 w459] -> w444
              tunnel: w447 -> [w456 w458]
              tunnel: [w456 w458] -> w446
              frame Default {
              }
              frame "Error" {
                n218 = Variant To Data(type=errorcluster {"status"=FALSE, "code"=0, "source"=""} ("error constant"), Variant=w461) -> (data=w459:errorcluster)  [unwired: 1 in, 1 out]
              }
            }
            n219 = call "Dialog - Error Message.vi"("error in"=w444) -> ("Selection"=w448:enum16{"Exit", "Reset", "Ignore"})
            n220 = call <vilib>:"Event Log.Record Event.vi"("error in"=w444) -> ()  [unwired: 10 in, 1 out]
            n221 = case shown="\"Reset\"" w448 {
              tunnel: w446 -> [w453 _ w455]
              tunnel: [w452 _ w454] -> w445
              frame "Exit", Default {
                n222 = call <vilib>:"Q.Enqueue Exit.vi"("Q In"=w453) -> ("error out"=w452:errorcluster)  [unwired: 9 in, 1 out]
              }
              frame "Ignore" {
              }
              frame "Reset" {
                n223 = call <vilib>:"Q.Enqueue Reset.vi"("Q In"=w455) -> ("error out"=w454:errorcluster)  [unwired: 9 in, 1 out]
              }
            }
          }
          frame Default {
            n224 = Concatenate Strings("Undefined State: \"", w462, "\".") -> (w464:string)
            n225 = Bundle By Name(cluster=errorcluster {"status"=TRUE, "code"=-5000, "source"=""} ("error constant"), "source"=w464) -> (w463:errorcluster)
          }
        }
      }
      frame "Exit" {
        # "Save control states"
        n226 = Unbundle By Name(w469) -> ("Log.Open"=w474:bool, "Log.FileRef"=w475:refnum<k34>)
        n227 = case shown="True" w474 {
          tunnel: w475 -> [_ w479]
          tunnel: [_ w478] -> _
          frame False {
          }
          frame True {
            n228 = TDMS Close(11:w479) -> (0:w478:errorcluster)  [unwired: 1 in, 1 out]
          }
        }
        n229 = Unbundle By Name(w471) -> ("Cfg.Dirs.App Data"=w468:path, "Cfg.Name"=w472:string)
        n230 = call "Save Control - Manager.vi"("App Data Dir"=w468, "Action"=Save_Control_-_Action."Save", "App Name"=w472) -> ("error out"=w470:errorcluster)  [unwired: 8 in]
        n231 = call <vilib>:"Clear Errors.vi"("error in (no error)"=w470) -> ()  [unwired: 5 in, 2 out]
        n232 = call <vilib>:"Module.Destructor.vi"("Sys"=w471) -> ("error out"=w477:errorcluster)  [unwired: 10 in]
      }
    }
  }
